vi "Path - When Constructed - Returns Configured Value.vi"() -> ()   [LabVIEW 2017, in "Test Case.Tests.lvlib"]
uses:
  Test Case.Tests.lvlib
  Test Case/Test Case.lvclass/Test Case.ctl
  fc41dd10-c4f1-4a55-a86a-822b6e90fa10.vi
  Test Case/Get Path.vi
  Constraint/IsEqual/Create.vi
  Constraint/IsEqual/IsEqual.lvclass
  Test Case/Test Case.lvclass
panel:
  out "error out":errorcluster
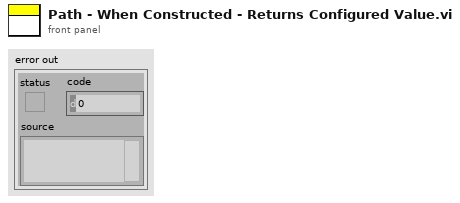
[diagram p1: front panel]
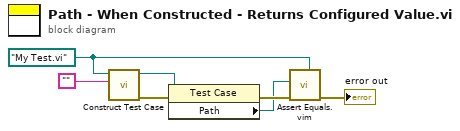
[diagram p0: block diagram]
diagram:
  w2 = path "My Test.vi" ("Path")
  n1 = call "Construct Test Case.vi"("Qualified Name"="", "Path"=w2) -> ("error out"=w7:errorcluster, "Test Case"=w4:refnum<class "Test Case.lvclass">)  [unwired: 8 in]
  n2 = property class="Test Case"(reference=w4, error in=w7) -> (error out=w5:errorcluster, "Path"=w3:path)  [unwired: 1 out]
  n3 = call "Assert Equals.vim"("Expected"=w2, "error in (no error)"=w5, "Actual"=w3) -> ("error out"=→"error out":errorcluster)  [unwired: 8 in]
